vi "11.2.1.-Abrir y Binarizar Imagen.vi"() -> (0 "F":dbl[][](array[numeric]), 1 "Y":dbl[][](array[numeric]), 2 "X":dbl[][](array[numeric]), 4 "Imagen seleccionada":picture)   [LabVIEW 2020]
uses:
  <vilib>/Analysis/Matrix/Numeric/Conversions/Array To Matrix - RA2.vi
  <vilib>/Analysis/Matrix/Numeric/Conversions/Matrix To Array - RM.vi
  <vilib>/Analysis/Matrix/NI_Matrix.lvlib
panel:
  in  "File Path":path
  # "Visión Artificial - Momentos Invariantes de Hu\nDiego Cervantes Rodríguez\ndicer0.com"
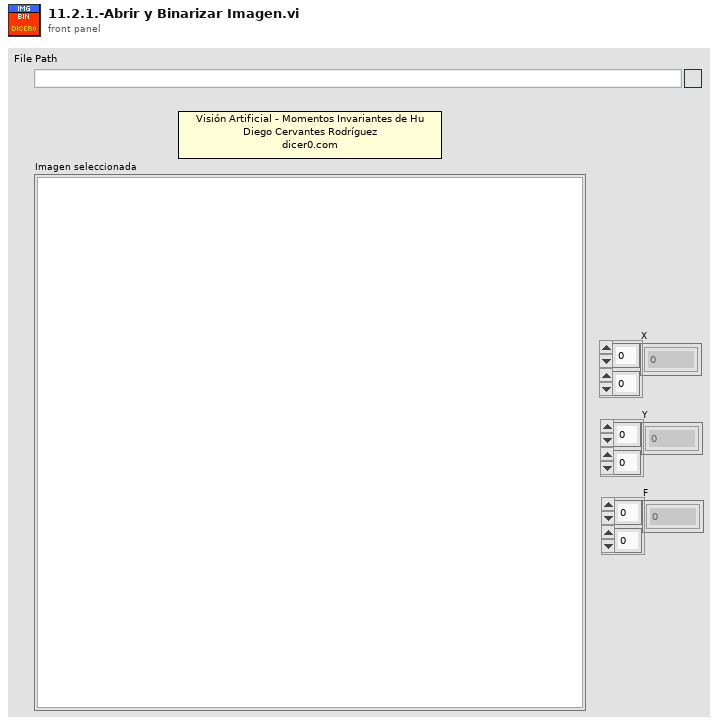
[diagram p1: front panel]
types:
  T1 = typedef "imagedata.ctl" = cluster{"image type":i32, "image depth":i32, "image":u8[], "mask":u8[], "colors":u32[], "Rectangle":cluster{"left":i16, "top":i16, "right":i16, "bottom":i16}}
  T2 = typedef "NI_Matrix.lvlib/RealMatrix.ctl" = dbl[][]
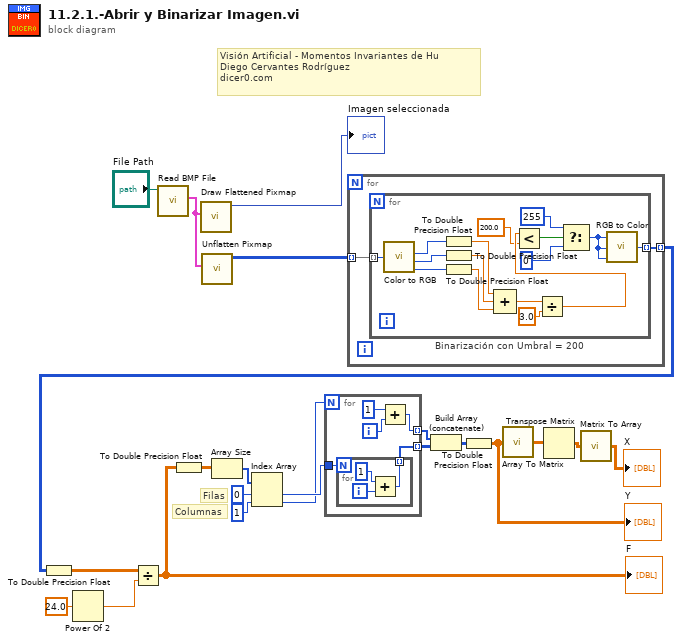
[diagram p0: block diagram]
diagram:
  # "Visión Artificial - Momentos Invariantes de Hu\nDiego Cervantes Rodríguez\ndicer0.com"
  # "Columnas"
  # "Filas"
  n1 = Power Of 2(x=24.0 ("y")) -> (2^x=w19:dbl)
  n2 = call <vilib>:"Read BMP File.vi"("path to BMP file"="File Path") -> ("image data"=w4:T1)  [unwired: 8 in, 2 out]
  n3 = call <vilib>:"Draw Flattened Pixmap.vi"("image data"=w4) -> ("new picture"=→"Imagen seleccionada":picture)  [unwired: 8 in]
  n4 = call <vilib>:"Unflatten Pixmap.vi"("image data"=w4) -> ("24-bit pixmap"=w22:u32[][])  [unwired: 4 in, 6 out]
  n5 = for {
    tunnel: w22 -> [w24] mode=indexing
    tunnel: [w23] -> w14 mode=indexing
    n6 = for "Binarización con Umbral = 200" {
      tunnel: w24 -> [w36] mode=indexing
      tunnel: [w32] -> w23 mode=indexing
      n7 = call <vilib>:"Color to RGB.vi"("Color"=w36) -> ("R"=w31:u8, "G"=w30:u8, "B"=w29:u8)  [unwired: 1 out]
      n8 = To Double Precision Float(number=w31) -> (double precision float=w28:dbl)
      n9 = To Double Precision Float(number=w30) -> (double precision float=w27:dbl)
      n10 = To Double Precision Float(number=w29) -> (double precision float=w26:dbl)
      n11 = Compound Arithmetic op=ADD(w28, w27, w26) -> (w25:dbl)
      n12 = Divide(x=w25, y=3.0) -> (x/y=w34:dbl)
      n13 = Less?(x=w34, y=200.0) -> (x < y?=w38:bool)
      n14 = Select(t=u8 255 ("y"), s=w38, f=u8 0 ("y")) -> (s? t:f=w37:u8)
      n15 = call <vilib>:"RGB to Color.vi"("B"=w37, "G"=w37, "R"=w37) -> ("Color"=w32:u32)
    }
  }
  n16 = To Double Precision Float(number=w14) -> (double precision float=w2:dbl[][])
  n17 = Divide(x=w2, y=w19) -> (x/y=w15:dbl[][])
  "F" <- w15
  n18 = To Double Precision Float(number=w15) -> (double precision float=w12:dbl[][])
  n19 = Array Size(array=w12) -> (size(s)=w13:i32[])
  n20 = Index Array "Index Array"(array=w13, index #1=0 ("index"), index #2=1 ("index")) -> (element #1=w9:i32, element #2=w8:i32)
  n21 = for {
    N: w8 -> [_]
    tunnel: [w41] -> w7 mode=indexing
    tunnel: w9 -> [w44]
    tunnel: [w43] -> w20 mode=indexing
    i -> [w42]
    n22 = for {
      N: w44 -> [_]
      tunnel: [w47] -> w43 mode=indexing
      i -> [w48]
      n23 = Add(x=1, y=w48) -> (x+y=w47:i32)
    }
    n24 = Add(x=1, y=w42) -> (x+y=w41:i32)
  }
  n25 = Build Array (concatenate) "Build Array"(w7, w20) -> (w21:i32[][])
  n26 = To Double Precision Float(number=w21) -> (double precision float=w17:dbl[][])
  "Y" <- w17
  n27 = call-poly <vilib>:"Array To Matrix.vi"("Real 2D Array"=w17) -> ("Real Matrix"=w10:T2)
  n28 = Transpose Matrix(1:w10) -> (0:w11:T2)
  n29 = call-poly <vilib>:"Matrix To Array.vi"("Real Matrix"=w11) -> ("Real 2D Array"=→"X":dbl[][])
